vi "AddUpdateEvent.vi"(8 "error in (no error)":errorcluster, 10 "UpdateEvent":refnum<user-event>, 11 "reference in":refnum<class "Switch_Manager.lvclass">) -> (0 "error out":errorcluster, 3 "reference in":refnum<class "Switch_Manager.lvclass">)   [LabVIEW 2022 SP3, in "Switch_Manager.lvlib" / "Switch_Manager.lvclass"]
uses:
  Switch_Manager.lvclass
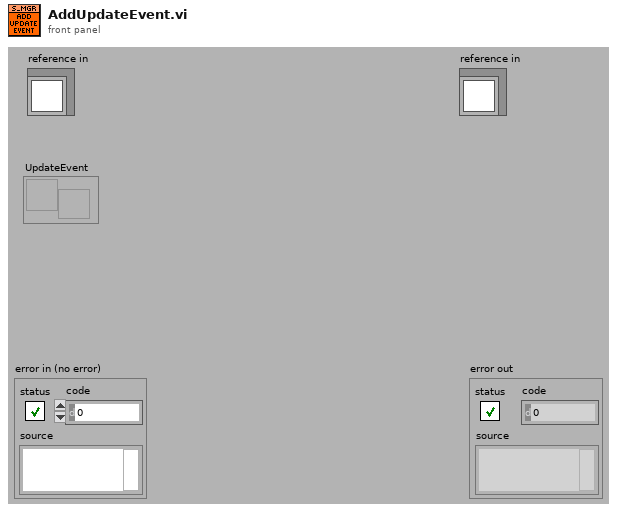
[diagram p1: front panel]
types:
  T1 = typedef "Switch_Manager.lvlib/Switch_Manager.lvclass/ObjectAttributes.ctl" = cluster{"Config":T2, "State":bool[], "Switches":refnum<class "SwitchBase.lvclass">[], "SwitchName":string[], "SwitchMap":T3[], "UpdateEvent":refnum<user-event>, "ParentEvent":refnum<user-event>, "Tree":bool[]}
  T2 = typedef "Switch_Manager.lvlib/Switch_Manager.lvclass/Config.ctl" = cluster{"default":string}
  T3 = typedef "Switch_Manager.lvlib/Switch_Manager.lvclass/SwitchMap.ctl" = cluster{"Name":string, "Description":string, "Group":string, "IsGroup":bool, "Switches":string[]}
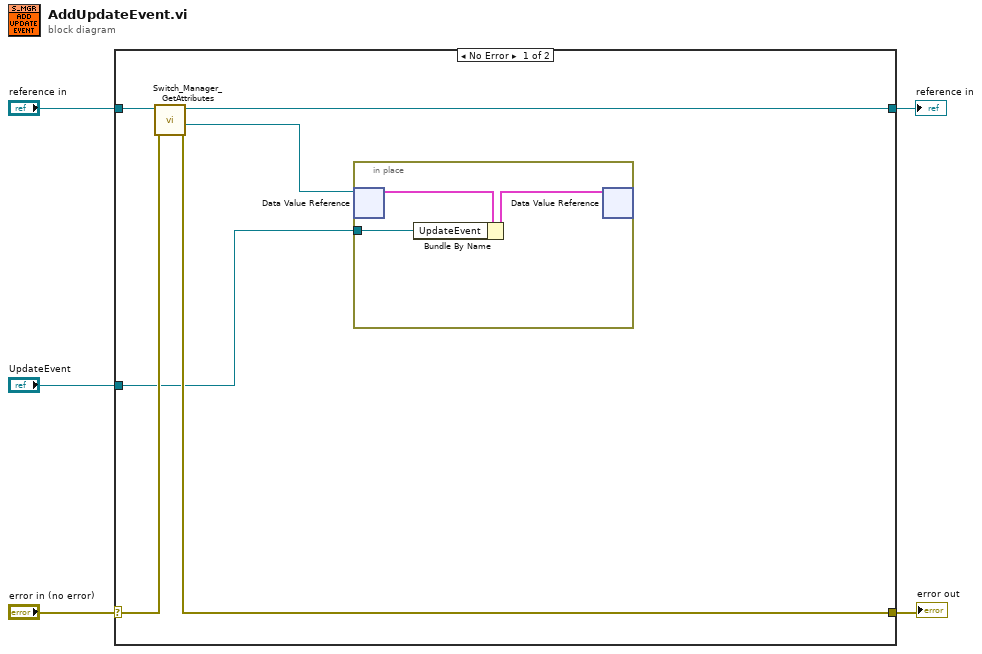
[diagram p0: block diagram]
diagram:
  n1 = case shown="No Error" "error in (no error)" {
    selector: "error in (no error)" -> [w11 w16]
    tunnel: [w10 w16] -> w4
    tunnel: [w8 w15] -> w2
    tunnel: "reference in" -> [w9 w15]
    tunnel: "UpdateEvent" -> [w6 _]
    frame No Error {
      n2 = call "Switch_Manager_GetAttributes.vi"("error in (no error)"=w11, "reference in"=w9) -> ("error out"=w10:errorcluster, "DataRef"=w7:refnum<data-value>, "reference out"=w8:refnum<class "Switch_Manager.lvclass">)  [unwired: 6 in, 1 out]
      n3 = in-place {
        in-place-border: w6 -> [w12]
        n4 = in-place-dvr #1(w7) -> (w14:T1)  [unwired: 1 out]
        n5 = Bundle By Name(cluster=w14, "UpdateEvent"=w12) -> (w13:T1)
        n6 = in-place-dvr #1(w13) -> ()  [unwired: 2 out]
      }
    }
    frame Error {
    }
  }
  "error out" <- w4
  "reference in" <- w2
